vi "Invite.vi"(9 "Convidar":bool, 11 "DataIn":T5) -> (3 "Data out":T1)   [LabVIEW 2017]
uses:
  controls/DataIn.ctl
  controls/Tabuleiro.ctl
  controls/GameOption.ctl
  controls/Table.ctl
  controls/DataOut.ctl
  <userlib>/_SmartBalloon/API/SmartBalloon Library.lvclass/SmartBalloon Library.ctl
  <userlib>/_SmartBalloon/Balloon Generic/Balloon.lvclass/Balloon.ctl
  <userlib>/_SmartBalloon/Balloon Generic/Aesthetics.ctl
  <userlib>/_SmartBalloon/Balloon Generic/Read Text.vi
  <userlib>/_SmartBalloon/API/Read Events.vi
  <userlib>/_SmartBalloon/Balloon/Text Balloon.lvclass
  C:/Program Files (x86)/National Instruments/LabVIEW 2017/user.lib/_SmartBalloon/Balloon Generic/Balloon.lvclass
  <userlib>/_SmartBalloon/Balloon Generic/Balloon.lvclass
  <userlib>/_SmartBalloon/API/SmartBalloon Library.lvclass
panel:
  out "Click Time Stamp":timestamp
  out "Clicked Balloon Title":string
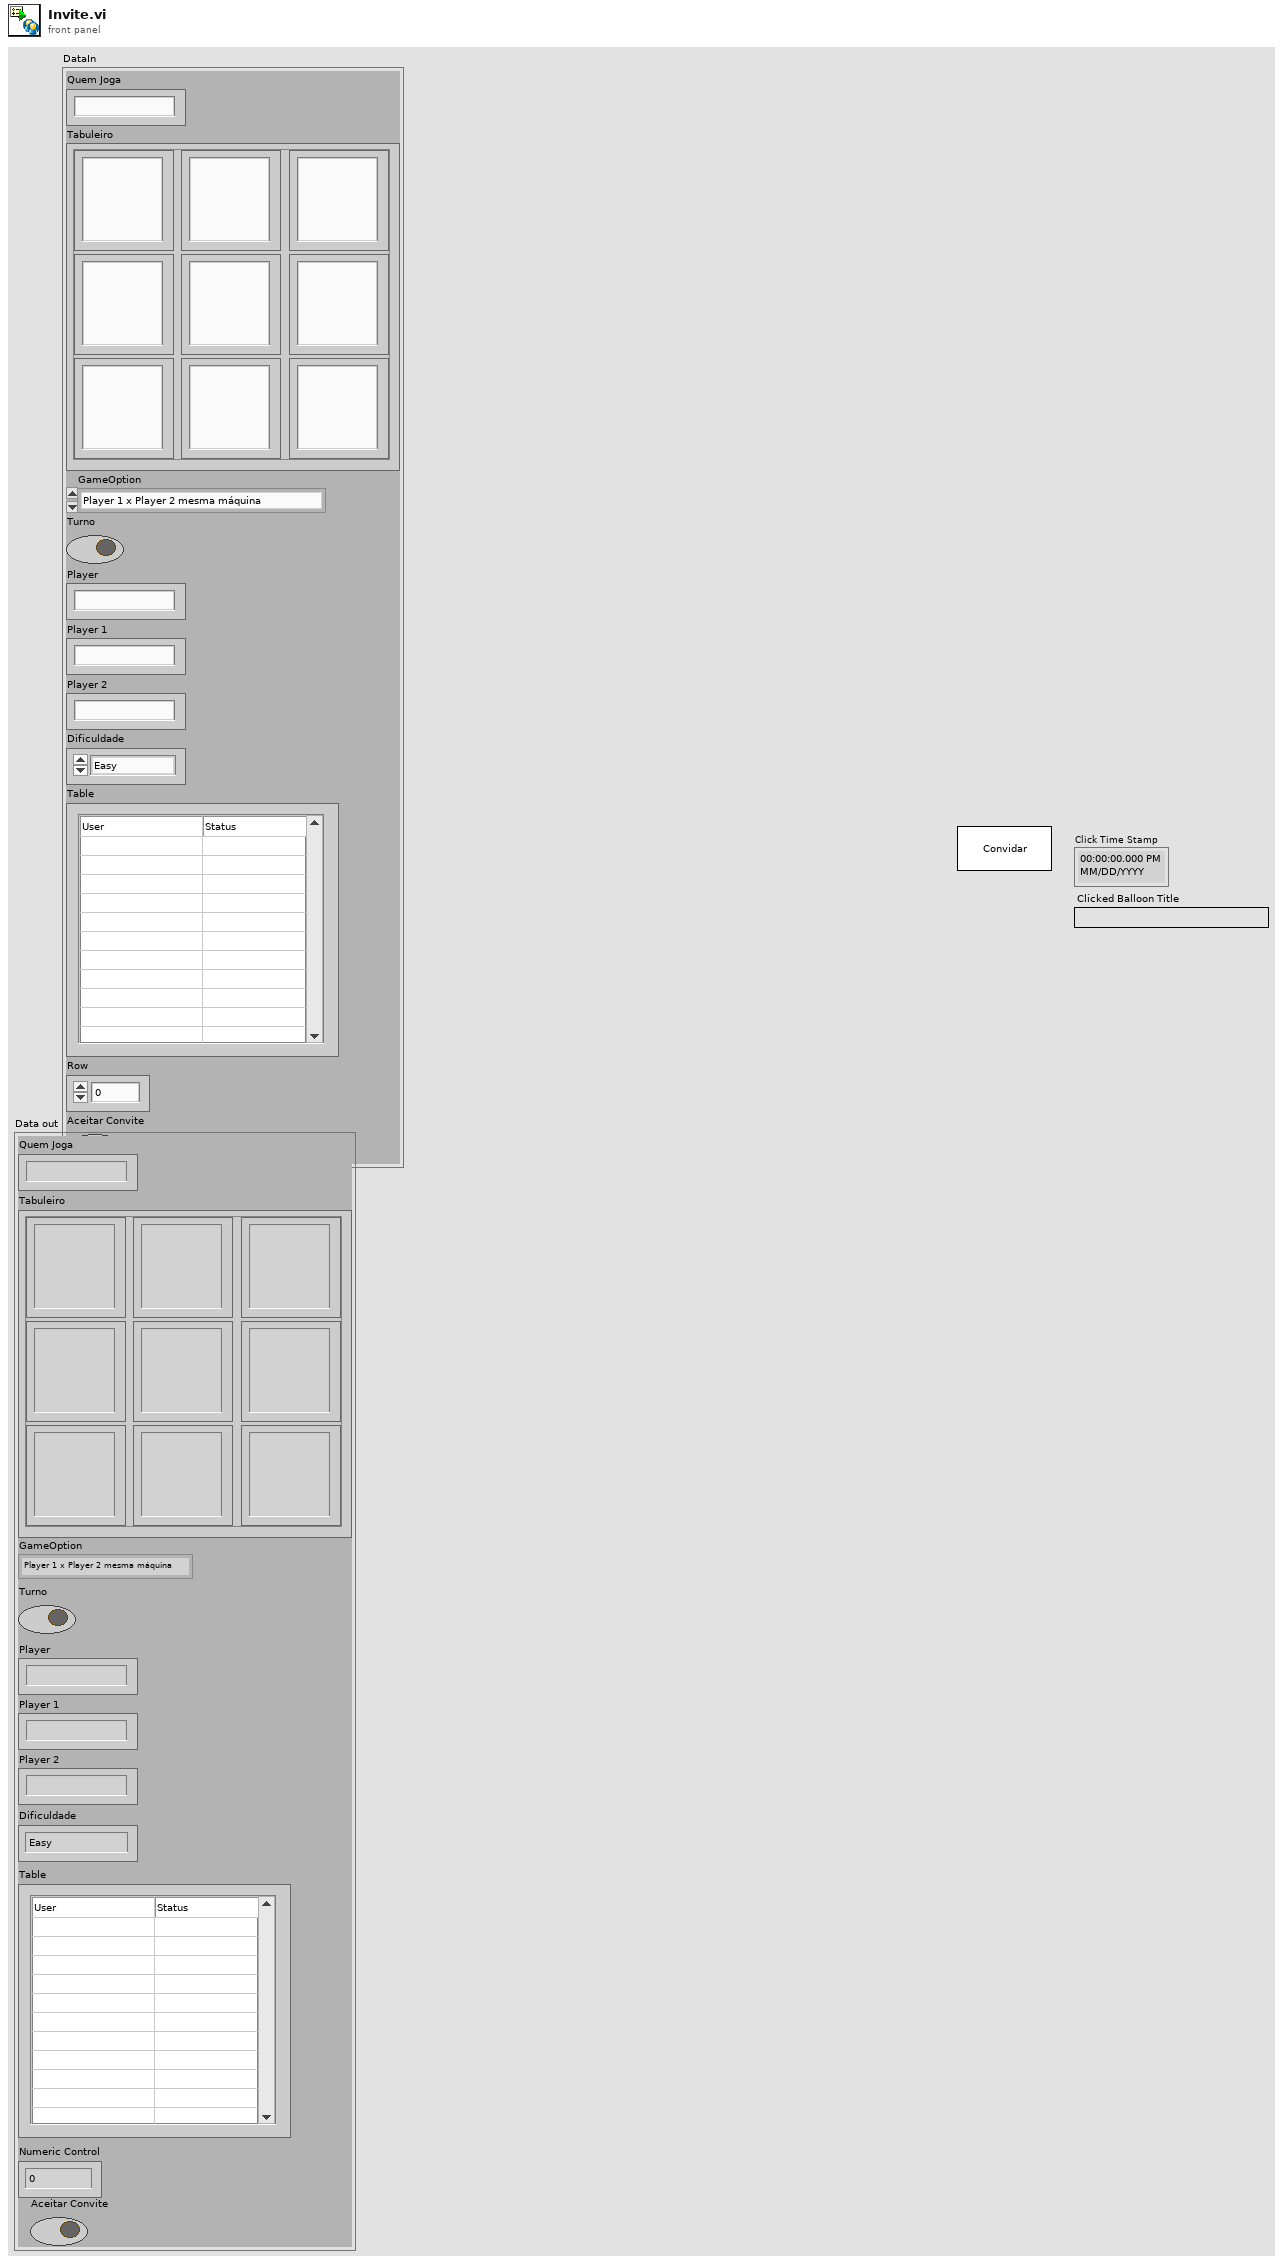
[diagram p1: front panel]
types:
  T1 = typedef "DataOut.ctl" = cluster{"Quem Joga":string, "Tabuleiro":T2, "GameOption":T3, "Turno":bool, "Player":string, "Player 1":string, "Player 2":string, "Dificuldade":enum16{"Easy", "Medium", "Hard"}, "Table":T4, "Numeric Control":u32, "Aceitar Convite":bool}
  T2 = typedef "Tabuleiro.ctl" = cluster{"(0,0)":string, "(1,0)":string, "(0,1)":string, "(1,1)":string, "(2,0)":string, "(1,2)":string, "(2,2)":string, "(0,2)":string, "(2,1) ":string}
  T3 = typedef "GameOption.ctl" = enum16{"Player 1 x Player 2 mesma máquina", "Player 1 x Player 2 pela rede", "Player 1 x Computador", "Wait for Event", "Initialize", "Stop"}
  T4 = typedef "Table.ctl" = string[][]
  T5 = typedef "DataIn.ctl" = cluster{"Quem Joga":string, "Tabuleiro":T2, "GameOption":T3, "Turno":bool, "Player":string, "Player 1":string, "Player 2":string, "Dificuldade":enum16{"Easy", "Medium", "Hard"}, "Table":T4, "Row":u32, "Aceitar Convite":bool}
  T6 = typedef "Balloon Engine.lvlib/Balloon Display Controller.lvclass/Controller Events.ctl" = cluster{"BalloonError Event":refnum<user-event>, "BalloonClicked Event":refnum<user-event>}
  T7 = typedef "Balloon Engine.lvlib/Balloon.lvclass/Aesthetics.ctl" = cluster{"Colors":cluster{"Font Color":u32, "Panel Color":u32}, "Display Time (ms)":i32}
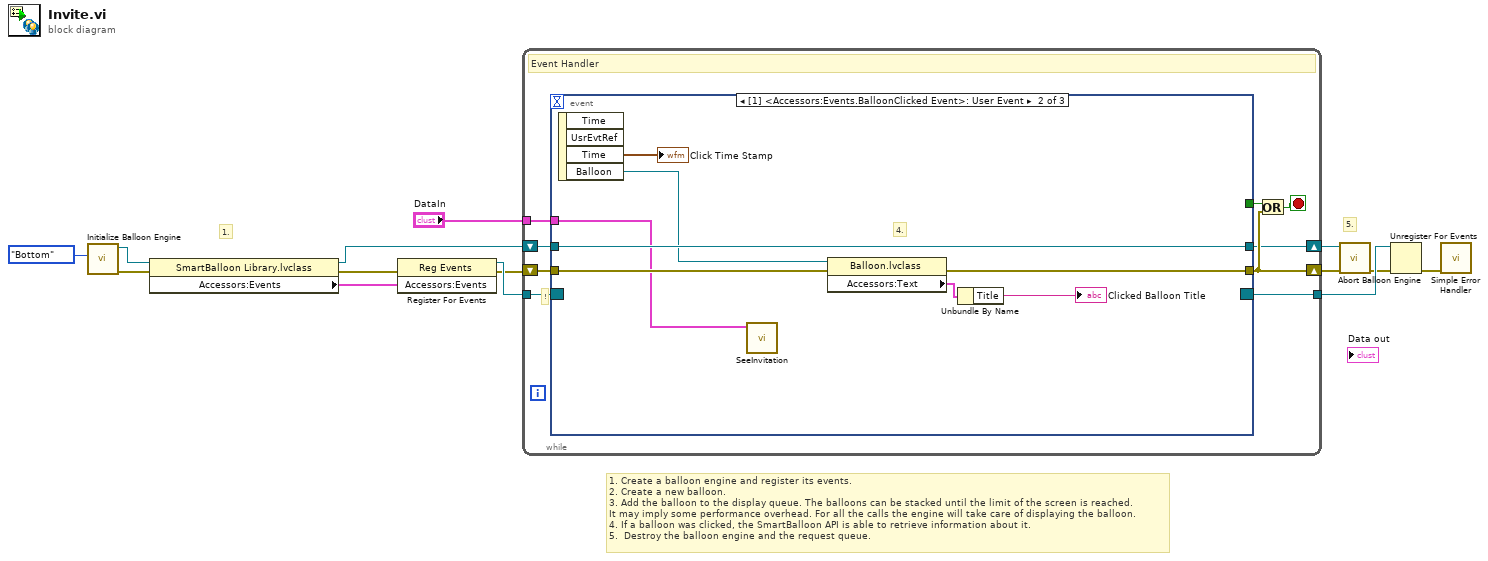
[diagram p0: block diagram]
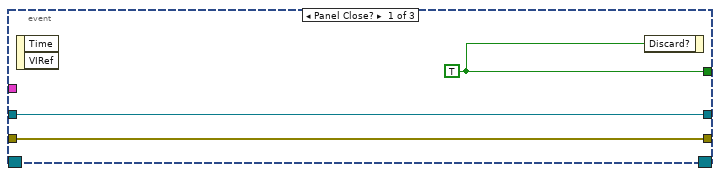
[diagram p2: hidden frame]
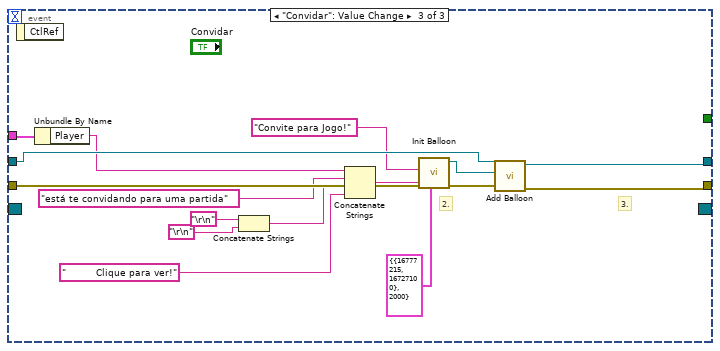
[diagram p3: hidden frame]
diagram:
  # "5."
  # "1."
  # "1. Create a balloon engine and register its events.\n2. Create a new balloon.\n3. Add the balloon to the display queue. The balloons can be stacked until the limit of the screen is reached. \nIt may imply some performance overhead. For all the calls the engine will take care of displaying the balloon.\n4. If a balloon was clicked, the SmartBalloon API is able to retrieve information about it.\n5.  Destroy the balloon engine and the request queue."
  n1 = call <userlib>:"Initialize Balloon Engine.vi"("Balloon Direction"=enum16{"Top", "Bottom"}."Bottom" ("Balloon Position")) -> ("error out"=w12:errorcluster, "SmartBalloon Library.lvclass"=w10:refnum<class "SmartBalloon Library.lvclass">)  [unwired: 9 in]
  n2 = property class="SmartBalloon Library.lvclass"(reference=w10, error in=w12) -> (reference out=w14:refnum<class "SmartBalloon Library.lvclass">, error out=w13:errorcluster, "Accessors:Events"=w11:T6)
  n3 = register-events(error in=w13, w11) -> (reference out=w4:refnum<event-registration>, error out=w3:errorcluster)  [unwired: 1 in]
  n4 = while {
    shift-right: [w19] -> w5
    shift-left: w3 -> [w22]
    tunnel: w4 -> [w18]
    shift-right: [w17] -> w6
    shift-left: w14 -> [w21]
    tunnel: [w16] -> w9
    tunnel: "DataIn" -> [w15]
    stop <- w20 stop-if-true
    # "!"
    # "Event Handler"
    n5 = event shown="[1] <Accessors:Events.BalloonClicked Event>: User Event" {
      selector: w18 -> [_ _ _]
      dyn-events: [_ _ _] -> w16
      timeout: _ -> [_ _ _]
      tunnel: [w26 _ _] -> w23
      tunnel: [w25 w32 w39] -> w19
      tunnel: w22 -> [w25 w28 w50]
      tunnel: w21 -> [w24 w31 w48]
      tunnel: [w24 w31 w38] -> w17
      tunnel: w15 -> [_ w27 w43]
      event Panel Close? {
        w26 = TRUE ("Discard?")
        n6 = event-data() -> ()  [unwired: 1 in, 2 out]
        n7 = event-data("Discard?"=w26) -> ()  [unwired: 1 in, 1 out]
      }
      event User Event {
        # "4."
        n8 = event-data() -> ("Time"=→"Click Time Stamp":timestamp, "Balloon"=w29:refnum<class "Balloon.lvclass">)  [unwired: 1 in, 2 out]
        n9 = call "SeeInvitation.vi"("DataIn"=w27) -> ()  [unwired: 10 in, 1 out]
        n10 = property class="Balloon.lvclass"(reference=w29, error in=w28) -> (error out=w32:errorcluster, "Accessors:Text"=w34:cluster{"Title":string, "Body":string})  [unwired: 1 out]
        n11 = Unbundle By Name(w34) -> ("Title"=→"Clicked Balloon Title":string)
      }
      event "Convidar": Value Change {
        # "3."
        # "2."
        n12 = event-data() -> ()  [unwired: 1 in, 1 out]
        n13 = Unbundle By Name(w43) -> ("Player"=w42:string)
        n14 = Concatenate Strings("\r\n", "\r\n") -> (w36:string)
        n15 = Concatenate Strings(w42, "está te convidando para uma partida" ("Body"), w36, "          Clique para ver!" ("string")) -> (w45:string)
        n16 = call <userlib>:"Init Balloon.vi"("Aesthetics"=T7 {"Colors"={"Font Color"=16777215, "Panel Color"=16727100}, "Display Time (ms)"=2000} ("Balloon Settings"), "error in (no error)"=w50, "Body"=w45, "Title"="Convite para Jogo!") -> ("error out"=w47:errorcluster, "Balloon out"=w41:refnum<class "Text Balloon.lvclass">)  [unwired: 6 in]
        n17 = call <userlib>:"Add Balloon.vi"("error in (no error)"=w47, "Next Balloon"=w41, "SmartBalloon Engine Reference"=w48) -> ("error out"=w39:errorcluster, "SmartBalloon Engine Reference out"=w38:refnum<class "SmartBalloon Library.lvclass">)  [unwired: 7 in]
      }
    }
    n18 = Or(x=w23, y=w19) -> (x .or. y?=w20:bool)
  }
  n19 = call <userlib>:"Abort Balloon Engine.vi"("error in (no error)"=w5, "SmartBalloon Engine Reference"=w6) -> ("error out"=w7:errorcluster)  [unwired: 9 in]
  n20 = Unregister For Events(event registration refnum=w9, error in=w7) -> (error out=w8:errorcluster)
  n21 = call <vilib>:"Simple Error Handler.vi"("error in (no error)"=w8) -> ()  [unwired: 4 in, 5 out]
